vi "ImagesToAVI.vi"() -> ()   [LabVIEW 2012, in "HGF_VisionTools.lvlib"]
doc: "This VI can be used to create an AVI file from images located in one folder. Frame rate can be configured."
uses:
  HGF_VisionTools.lvlib
  <vilib>/vision/NI_Vision_Development_Module.lvlib
  UtilityLib/UtilityLib.lvlib
  UtilityLib/UtilityLib.helpType.ctl
panel:
  in  "Pattern":string
  out "Path":path
  in  "Convert":bool
  in  "File listbox":i32[](listbox)
  out "Progress":dbl(slide) scale=0.0..1.0
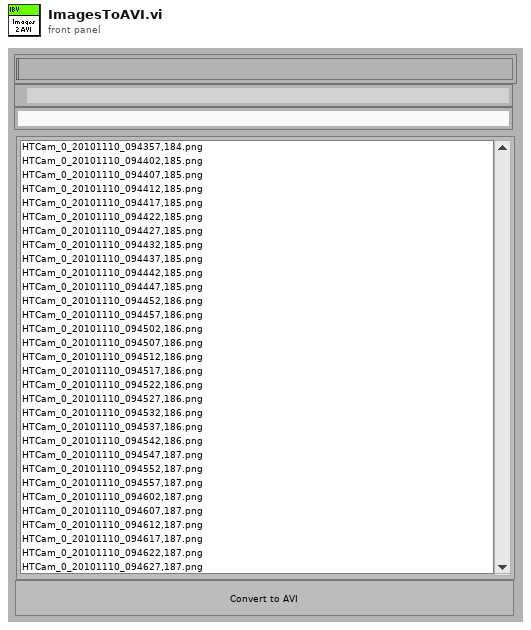
[diagram p1: front panel]
types:
  T1 = typedef "UtilityLib.lvlib/UtilityLib.helpType.ctl" = enum16{"unknown", "menu", "description", "about", "special0", "special1", "special2"}
  T2 = enum32{"invalid app kind", "Development System", "Run Time System", "Student Edition", "Embedded LabVIEW", "Evaluation", "Custom"}
  T3 = cluster{"Major":u16, "Minor":u16, "Fix":u16, "Build":u16}
  T4 = typedef "LVMenuShortCut.ctl" = cluster{"include Shift key?":bool, "include Ctrl key?":bool, "shortcut key":string}
  T5 = typedef "Image Type" = u32
  T6 = typedef "IMAQ Image.ctl" = refnum<image>
  T7 = typedef "AviRefnum.ctl" = refnum<k1>
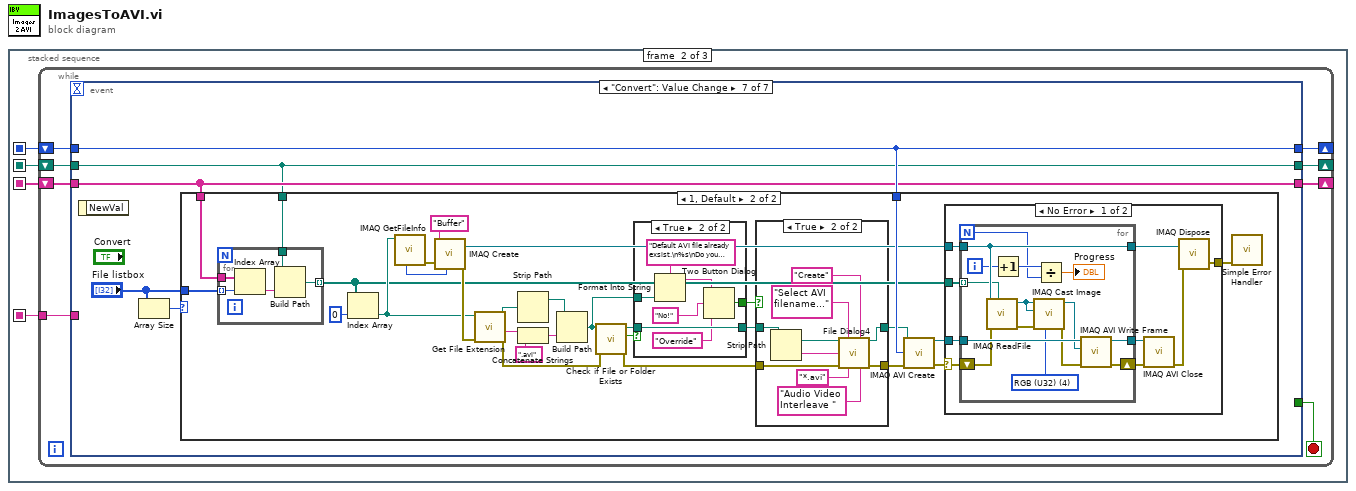
[diagram p0: block diagram]
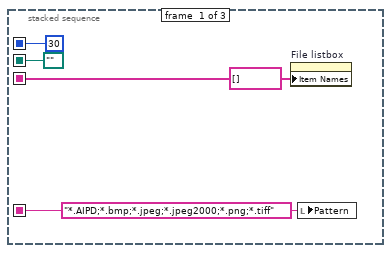
[diagram p2: hidden frame]
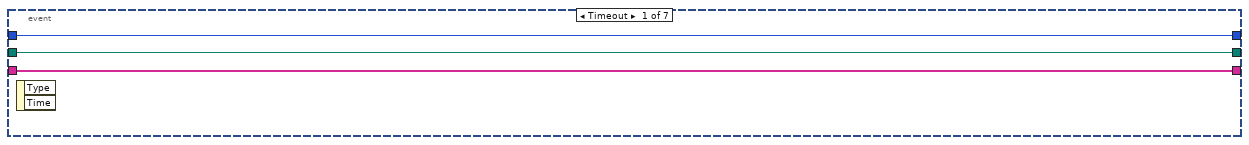
[diagram p3: hidden frame]
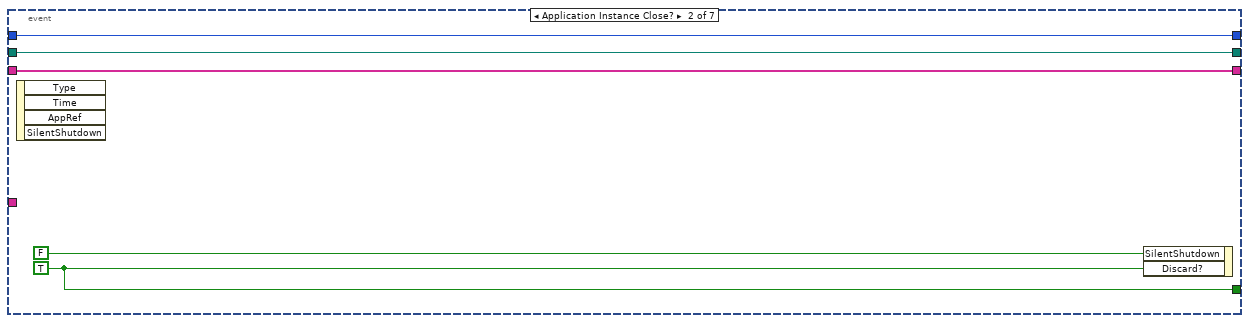
[diagram p4: hidden frame]
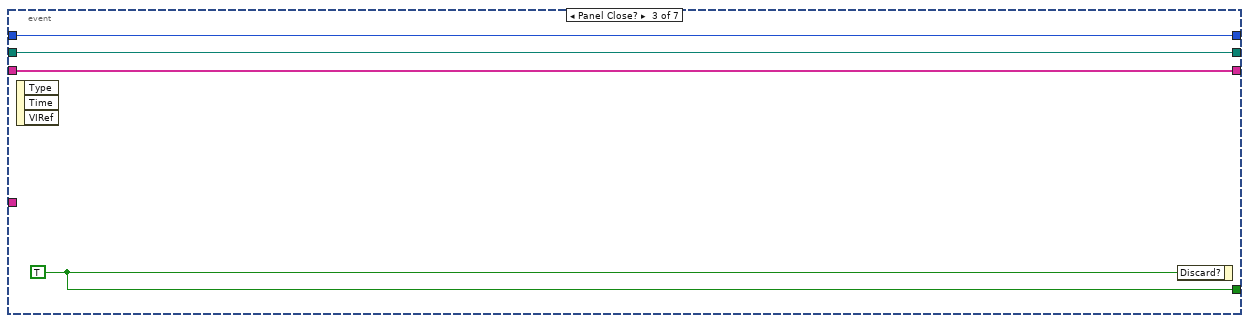
[diagram p5: hidden frame]
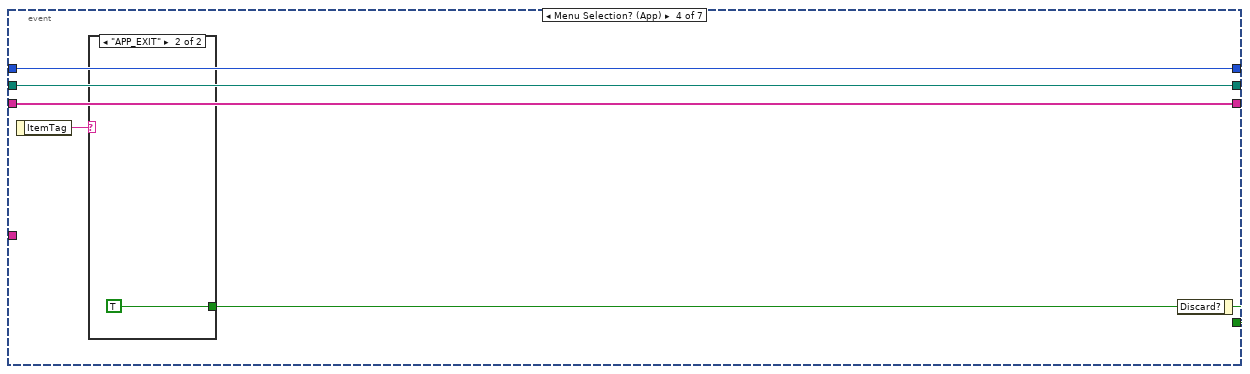
[diagram p6: hidden frame]
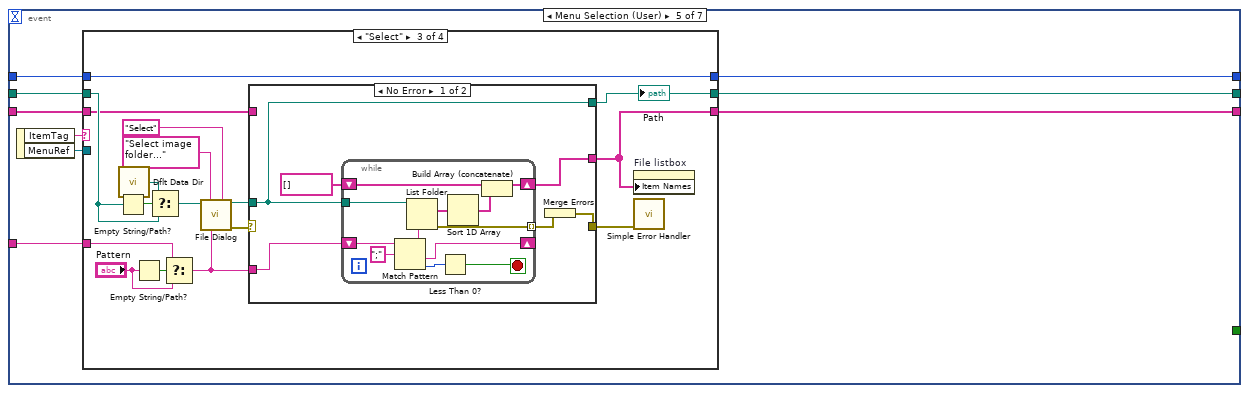
[diagram p8: hidden frame]
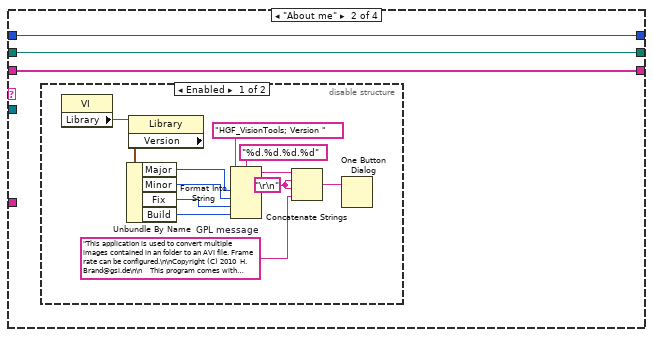
[diagram p10: hidden frame]
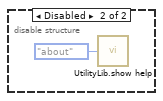
[diagram p11: hidden frame]
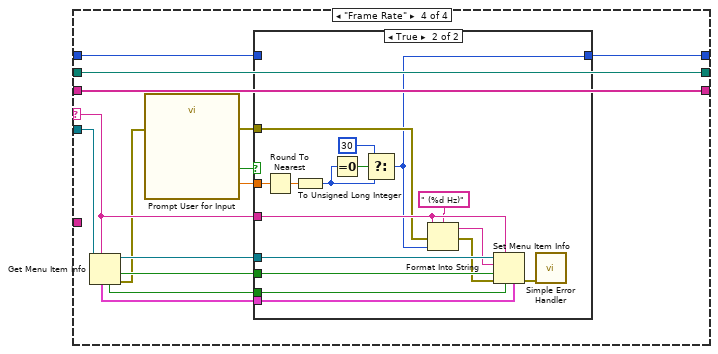
[diagram p13: hidden frame]
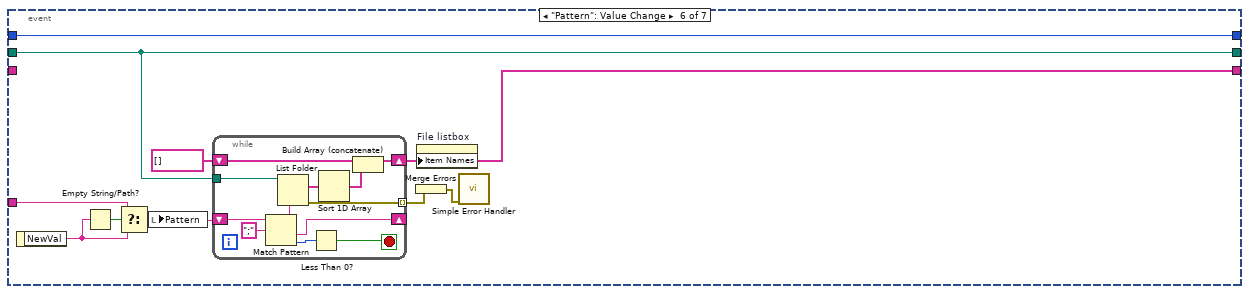
[diagram p15: hidden frame]
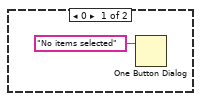
[diagram p16: hidden frame]
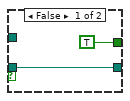
[diagram p18: hidden frame]
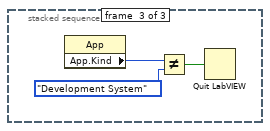
[diagram p20: hidden frame]
diagram:
  n1 = stacked-sequence {
    seq-local: [w4 _ _] -> [_ w8 _]
    seq-local: [w1 _ _] -> [_ w7 _]
    seq-local: [path "" _ _] -> [_ w6 _]
    seq-local: [u32 30 _ _] -> [_ w5 _]
    frame #0 {
      w4 = "*.AIPD;*.bmp;*.jpeg;*.jpeg2000;*.png;*.tiff" ("pattern (all files)")
      w1 = string[] [] ("Item Names")
      n2 = property on="File listbox" class="LstBox (strict)"("Item Names"=w1) -> ()  [unwired: 2 in, 2 out]
      n3 = local write "Pattern"(w4) -> ()
    }
    frame #1 {
      n4 = while {
        shift-right: [w15] -> _
        shift-left: w6 -> [w14]
        shift-right: [w13] -> _
        shift-left: w5 -> [w12]
        shift-right: [w11] -> _
        shift-left: w7 -> [w10]
        tunnel: w8 -> [w9]
        stop <- w16 stop-if-true
        n5 = event shown="[6] \"Convert\": Value Change" {
          selector: _ -> [_ _ _ _ _ _ _]
          dyn-events: _ -> [_ _ _ _ _ _ _]
          timeout: _ -> [_ _ _ _ _ _ _]
          tunnel: [_ w23 w28 w32 _ _ _] -> w16
          tunnel: [w19 w22 w27 w31 w42 w135 w156] -> w15
          tunnel: w14 -> [w19 w22 w27 w31 w41 w135 w156]
          tunnel: [w18 w21 w26 w30 w40 w141 w158] -> w13
          tunnel: w12 -> [w18 w21 w26 w30 w39 w141 w158]
          tunnel: [w17 w20 w25 w29 w37 w132 w157] -> w11
          tunnel: w10 -> [w17 w20 w25 w29 w36 _ w157]
          tunnel: w9 -> [_ _ _ _ w35 w140 _]
          event Timeout {
            n6 = event-data() -> ()  [unwired: 1 in, 2 out]
          }
          event Application Instance Close? {
            w23 = TRUE ("Discard?")
            n7 = event-data() -> ()  [unwired: 1 in, 4 out]
            n8 = event-data("SilentShutdown"=FALSE, "Discard?"=w23) -> ()  [unwired: 1 in, 1 out]
          }
          event Panel Close? {
            w28 = TRUE ("Discard?")
            n9 = event-data() -> ()  [unwired: 1 in, 3 out]
            n10 = event-data("Discard?"=w28) -> ()  [unwired: 1 in, 1 out]
          }
          event Menu Selection? (App) {
            n11 = event-data() -> ("ItemTag"=w33:string)  [unwired: 1 in]
            n12 = case shown="\"APP_EXIT\"" w33 {
              tunnel: [_ TRUE ("Discard?")] -> w32
              frame Default {
              }
              frame "APP_EXIT" {
              }
            }
            n13 = event-data("Discard?"=w32) -> ()  [unwired: 1 in, 1 out]
          }
          event Menu Selection (User) {
            n14 = event-data() -> ("ItemTag"=w43:string, "MenuRef"=w38:refnum<k9>)  [unwired: 1 in]
            n15 = case shown="\"Select\"" w43 {
              selector: w43 -> [_ _ _ w107]
              tunnel: [w46 w49 w67 w114] -> w42
              tunnel: w41 -> [w46 w49 w74 w114]
              tunnel: [w45 w48 w73 w106] -> w40
              tunnel: w39 -> [w45 w48 w73 w102]
              tunnel: w38 -> [_ _ _ w112]
              tunnel: [w44 w47 w68 w101] -> w37
              tunnel: w36 -> [w44 w47 w69 w101]
              tunnel: w35 -> [_ _ w63 _]
              frame Default {
              }
              frame "About me" {
                n16 = disable-structure shown="Enabled" {
                  frame Enabled {
                    w51 = "\r\n"
                    w53 = "This application is used to convert multiple images contained in an folder to an AVI file. Frame rate can be configured.\n\nCopyright (C) 2010  H.Brand@gsi.de\n\n    This program comes with ABSOLUTELY NO WARRANTY; for details refer to the \"Gnu GPL V3.txt\" or \"Gnu GPL V3.doc\" included in the distribution.\n    \nThis is free software, and you are welcome to redistribute it\n    under certain conditions; for details refer to the \"Gnu GPL V3.txt\" or \"Gnu GPL V3.doc\" included in the distribution.\n"  # GPL message
                    n17 = property class="VI"() -> ("Library"=w50:refnum<vi>)  [unwired: 2 in, 2 out]
                    n18 = property class="Library"(reference=w50) -> ("Version"=w61:T3)  [unwired: 1 in, 2 out]
                    n19 = Unbundle By Name(w61) -> ("Major"=w59:u16, "Minor"=w58:u16, "Fix"=w57:u16, "Build"=w56:u16)
                    n20 = Format Into String(format string="%d.%d.%d.%d", initial string="HGF_VisionTools; Version ", w59, w58, w57, w56) -> (resulting string=w54:string)  [unwired: 1 in, 1 out]
                    n21 = Concatenate Strings(w54, w51, w51, w53) -> (w52:string)
                    n22 = One Button Dialog(message=w52) -> ()  [unwired: 1 in, 1 out]
                  }
                  frame Disabled {
                    n23 = call "UtilityLib.show help.vi"("helpType"=UtilityLib.helpType."about") -> ()
                  }
                }
              }
              frame "Select" {
                n24 = Empty String/Path?(string/path=w74) -> (empty?=w77:bool)
                n25 = call <vilib>:"Dflt Data Dir.vi"() -> ("App:Default Data Directory"=w76:path)
                n26 = Empty String/Path?(string/path="Pattern") -> (empty?=w66:bool)
                n27 = Select(t=w76, s=w77, f=w74) -> (s? t:f=w75:path)
                n28 = Select(t=w63, s=w66, f="Pattern") -> (s? t:f=w65:string)
                n29 = call "File Dialog"("start path"=w75, "prompt"="Select image folder...", "button label"="Select", "pattern (all files)"=w65) -> ("selected path"=w71:path, "error out"=w70:errorcluster)  [unwired: 8 in, 2 out]
                n30 = case shown="No Error" w70 {
                  selector: w70 -> [_ w99]
                  tunnel: [w81 w99] -> w72
                  tunnel: w71 -> [w83 w100]
                  tunnel: [w83 w100] -> w67
                  tunnel: [w84 w98] -> w68
                  tunnel: w69 -> [_ w98]
                  tunnel: w65 -> [w80 _]
                  frame No Error {
                    n31 = while {
                      shift-right: [w96] -> _
                      shift-left: w80 -> [w97]
                      shift-right: [w89] -> w84
                      shift-left: string[] [] -> [w88]
                      tunnel: w83 -> [w87]
                      tunnel: [w86] -> w82 mode=indexing
                      stop <- w94 stop-if-true
                      n32 = Match Pattern(string=w97, regular expression=";") -> (before substring=w92:string, after substring=w96:string, offset past match=w93:i32)  [unwired: 1 in, 1 out]
                      n33 = List Folder(path=w87, pattern=w92) -> (filenames=w91:string[], error out=w86:errorcluster)  [unwired: 2 in, 2 out]
                      n34 = Less Than 0?(x=w93) -> (x < 0?=w94:bool)
                      n35 = Sort 1D Array(array=w91) -> (sorted array=w90:string[])
                      n36 = Build Array (concatenate)(w88, w90) -> (w89:string[])
                    }
                    n37 = Merge Errors(w82) -> (w81:errorcluster)
                  }
                  frame Error {
                  }
                }
                "Path" <- w67
                n38 = property on="File listbox" class="LstBox (strict)"("Item Names"=w68) -> ()  [unwired: 2 in, 2 out]
                n39 = call <vilib>:"Simple Error Handler.vi"("error in (no error)"=w72) -> ()  [unwired: 4 in, 5 out]
              }
              frame "Frame Rate" {
                n40 = Get Menu Item Info(7:w107, 11:w112) -> (0:w104:errorcluster, 1:w110:bool, 3:w111:refnum<k9>, 4:w109:bool, 6:w108:T4)  [unwired: 1 in, 2 out]
                n41 = call "Prompt User for Input"("error in (no error)"=w104) -> ("Frame Rate"=w113:dbl, "OK"=w103:bool, "error out"=w105:errorcluster)  [unwired: 16 in]
                n42 = case shown="True" w103 {
                  tunnel: w113 -> [_ w131]
                  tunnel: w111 -> [_ w129]
                  tunnel: w110 -> [_ w128]
                  tunnel: w109 -> [_ w127]
                  tunnel: w108 -> [_ w126]
                  tunnel: w107 -> [_ w125]
                  tunnel: [w115 w117] -> w106
                  tunnel: w105 -> [_ w123]
                  tunnel: w102 -> [w115 _]
                  frame False {
                  }
                  frame True {
                    n43 = Round To Nearest(number=w131) -> (nearest integer value=w130:dbl)
                    n44 = To Unsigned Long Integer(number=w130) -> (unsigned 32bit integer=w118:u32)
                    n45 = Equal To 0?(x=w118) -> (x = 0?=w119:bool)
                    n46 = Select(t=u32 30, s=w119, f=w118) -> (s? t:f=w117:u32)
                    n47 = Format Into String(format string=" (%d Hz)", initial string=w125, error in=w123, w117) -> (resulting string=w124:string, error out=w122:errorcluster)
                    n48 = Set Menu Item Info(4:w126, 6:w127, 7:w125, 8:w122, 9:w128, 10:w124, 11:w129) -> (0:w120:errorcluster)  [unwired: 1 out]
                    n49 = call <vilib>:"Simple Error Handler.vi"("error in (no error)"=w120) -> ()  [unwired: 4 in, 5 out]
                  }
                }
              }
            }
          }
          event "Pattern": Value Change {
            n50 = event-data() -> ("NewVal"=w139:string)  [unwired: 1 in]
            n51 = Empty String/Path?(string/path=w139) -> (empty?=w138:bool)
            n52 = Select(t=w140, s=w138, f=w139) -> (s? t:f=w134:string)
            n53 = local write "Pattern"(w134) -> ()
            n54 = while {
              shift-right: [w152] -> _
              shift-left: w134 -> [w153]
              shift-right: [w145] -> w132
              shift-left: string[] [] -> [w144]
              tunnel: w135 -> [w143]
              tunnel: [w142] -> w136 mode=indexing
              stop <- w150 stop-if-true
              n55 = Match Pattern(string=w153, regular expression=";") -> (before substring=w148:string, after substring=w152:string, offset past match=w149:i32)  [unwired: 1 in, 1 out]
              n56 = List Folder(path=w143, pattern=w148) -> (filenames=w147:string[], error out=w142:errorcluster)  [unwired: 2 in, 2 out]
              n57 = Less Than 0?(x=w149) -> (x < 0?=w150:bool)
              n58 = Sort 1D Array(array=w147) -> (sorted array=w146:string[])
              n59 = Build Array (concatenate)(w144, w146) -> (w145:string[])
            }
            n60 = Merge Errors(w136) -> (w133:errorcluster)
            n61 = property on="File listbox" class="LstBox (strict)"("Item Names"=w132) -> ()  [unwired: 2 in, 2 out]
            n62 = call <vilib>:"Simple Error Handler.vi"("error in (no error)"=w133) -> ()  [unwired: 4 in, 5 out]
          }
          event "Convert": Value Change {
            n63 = event-data() -> ()  [unwired: 1 in, 1 out]
            n64 = Array Size(array="File listbox") -> (size(s)=w155:i32)
            n65 = case shown="1, Default" w155 {
              tunnel: w158 -> [_ w188]
              tunnel: w157 -> [_ w165]
              tunnel: w156 -> [_ w164]
              tunnel: "File listbox" -> [_ w163]
              frame 0 {
                n66 = One Button Dialog(message="No items selected") -> ()  [unwired: 1 in, 1 out]
              }
              frame 1, Default {
                n67 = for {
                  tunnel: w165 -> [w193]
                  tunnel: w163 -> [w192] mode=indexing
                  tunnel: w164 -> [w190]
                  tunnel: [w189] -> w162 mode=indexing
                  n68 = Index Array(array=w193, index=w192) -> (element=w191:string)
                  n69 = Build Path(base path=w190, name or relative path=w191) -> (appended path=w189:path)
                }
                n70 = Index Array(array=w162, index=0) -> (element=w166:path)
                n71 = call "IMAQ GetFileInfo"("File Path"=w166) -> ("error out"=w179:errorcluster, "Image Type"=w180:T5)  [unwired: 4 in, 5 out]
                n72 = call "IMAQ Create"("Image Name"="Buffer", "Image Type"=w180, "error in (no error)"=w179) -> ("New Image"=w177:T6, "error out"=w178:errorcluster)  [unwired: 2 in]
                n73 = call <vilib>:"Get File Extension.vi"("error in (no error)"=w178, "file"=w166) -> ("error out"=w173:errorcluster, "filename without extension"=w183:string, "dup file"=w175:path)  [unwired: 6 in, 1 out]
                n74 = Strip Path(path=w175) -> (stripped path=w174:path)  [unwired: 1 out]
                n75 = Concatenate Strings(w183, ".avi" ("string")) -> (w181:string)
                n76 = Build Path(base path=w174, name or relative path=w181) -> (appended path=w160:path)
                n77 = call <vilib>:"Check if File or Folder Exists.vi"("error in (no error)"=w173, "path"=w160) -> ("error out"=w168:errorcluster, "file or folder exists?"=w172:bool, "dup path"=w171:path)  [unwired: 7 in]
                n78 = case shown="True" w172 {
                  tunnel: w171 -> [w207 w214]
                  tunnel: [w207 w214] -> w169
                  tunnel: [TRUE ("T button?") w213] -> w161
                  tunnel: w160 -> [_ w208]
                  frame False {
                  }
                  frame True {
                    n79 = Format Into String(format string="Default AVI file already exsist.\n%s\nDo you want to override?" ("message"), w208) -> (resulting string=w209:string)  [unwired: 2 in, 1 out]
                    n80 = Two Button Dialog(message=w209, 1:"Override" ("T button name (\"OK\")"), 2:"No!" ("F button name (\"Cancel\")")) -> (T button?=w213:bool)
                  }
                }
                n81 = case shown="True" w161 {
                  tunnel: [w195 w196] -> w170
                  tunnel: w169 -> [w195 w201]
                  tunnel: w168 -> [w194 w205]
                  tunnel: [w194 w204] -> w167
                  frame False {
                  }
                  frame True {
                    n82 = Strip Path(path=w201) -> (stripped path=w199:path, name=w200:string)
                    n83 = call "File Dialog4"("start path"=w199, "prompt"="Select AVI filename...", "button label"="Create", "default name"=w200, "error in"=w205, "pattern (all files)"="*.avi", "pattern label"="Audio Video Interleave ") -> ("selected path"=w196:path, "error out"=w204:errorcluster)  [unwired: 5 in, 2 out]
                  }
                }
                n84 = call "IMAQ AVI Create"("error in (no error)"=w167, "Frames Per Second"=w188, "AVI Path"=w170) -> ("error out"=w184:errorcluster, "Avi Refnum"=w185:T7)  [unwired: 7 in]
                n85 = case shown="No Error" w184 {
                  selector: w184 -> [w221 w239]
                  tunnel: w162 -> [w223 _]
                  tunnel: w185 -> [w222 _]
                  tunnel: [w215 w239] -> w187
                  tunnel: w177 -> [w218 _]
                  frame No Error {
                    n86 = for {
                      N -> [w226]
                      tunnel: w223 -> [w229] mode=indexing
                      tunnel: w222 -> [w238]
                      shift-right: [w237] -> w220
                      shift-left: w221 -> [w235]
                      tunnel: [w236] -> w219
                      tunnel: w218 -> [w234]
                      tunnel: [w234] -> w217
                      i -> [w227]
                      w225 = T5 4 items=["Grayscale (U8)", "Grayscale (I16)", "Grayscale (SGL)", "Complex (CSG)", "RGB (U32)", "HSL (U32)", "RGB (U64)", "Grayscale (U16)"] ("Image Type")
                      n87 = call "IMAQ ReadFile"("File Path"=w229, "error in (no error)"=w235, "Image"=w234) -> ("error out"=w231:errorcluster, "Image Out"=w232:T6)  [unwired: 4 in, 3 out]
                      n88 = Increment(x=w227) -> (x+1=w228:i32)
                      n89 = call "IMAQ Cast Image"("Image Type"=w225, "error in (no error)"=w231, "Image Dst"=w232, "Image Src"=w232) -> ("error out"=w230:errorcluster, "Image Dst Out"=w233:T6)  [unwired: 6 in]
                      n90 = Divide(x=w228, y=w226) -> (x/y=→"Progress":dbl)
                      n91 = call "IMAQ AVI Write Frame"("error in (no error)"=w230, "Image"=w233, "Avi Refnum"=w238) -> ("error out"=w237:errorcluster, "Avi Refnum (duplicate)"=w236:T7)  [unwired: 7 in]
                    }
                    n92 = call "IMAQ AVI Close"("error in (no error)"=w220, "Avi Refnum"=w219) -> ("error out"=w216:errorcluster)  [unwired: 9 in]
                    n93 = call "IMAQ Dispose"("Image"=w217, "error in (no error)"=w216) -> ("error out"=w215:errorcluster)  [unwired: 4 in]
                  }
                  frame Error {
                  }
                }
                n94 = call <vilib>:"Simple Error Handler.vi"("error in (no error)"=w187) -> ()  [unwired: 4 in, 5 out]
              }
            }
          }
        }
      }
    }
    frame #2 {
      n95 = property class="App"() -> ("App.Kind"=w240:T2)  [unwired: 2 in, 2 out]
      n96 = Not Equal?(x=w240, y=T2."Development System" ("Application:Kind")) -> (x != y?=w242:bool)
      n97 = Quit LabVIEW(quit? (T)=w242) -> ()
    }
  }
